vi "Receive Message.vi"(6 "priority":i32, 10 "Async Methods Actor in":refnum<class "Async Methods Actor.lvclass">, 11 "Message in":refnum<class "Message.lvclass">) -> (0 "error out":errorcluster, 2 "Async Actor out":refnum<class "Actor.lvclass">)   [LabVIEW 2023, in "Async Methods Actor.lvlib" / "Async Methods Actor.lvclass"]
doc: "This VI should be overriden ONLY if you are creating a proxy actor for remote transmission. If you are, override this VI to transmit the received message to a new destination, maintaining the given priority."
uses:
  Async Methods Actor.lvclass
  <vilib>/ActorFramework/Message/Message.lvclass
  <vilib>/ActorFramework/Actor/Actor.lvclass
  Async Methods Actor Messages/Async Message/Async Message.lvclass
  <vilib>/ActorFramework/Actor/Actor.lvclass/Actor.ctl
  <vilib>/ActorFramework/Message Enqueuer/Message Enqueuer.lvclass/Message Enqueuer.ctl
  Async Methods Actor.lvclass/Async Methods Actor.ctl
  Async Methods Actor Messages/Async Message/Async Message.lvclass/Async Message.ctl
  <vilib>/ActorFramework/Message Enqueuer/Init from Existing Queue.vi
  Add Async Message to Map.vi
  Async Methods Actor Messages/Async Message/Read Async Call Method.vi
  Async Methods Actor Messages/Async Message/Read VI Refnum Lifetime.vi
  Write Async Message Execution Status Map.vi
  Async Methods Actor Messages/Async Message/Read FQN.vi
  Write Async Message Execution Status Map.vi/3adbf29e-89d7-4ecb-a2bd-8a8b89d527f8.vi
  Get VI FQN.vi
  <vilib>/Utility/LVClass/Get LV Class Path.vi
  <vilib>/ActorFramework/Message Enqueuer/Message Enqueuer.lvclass
  <resource>/AFDebug/AF Debug.lvlib
  C:/Program Files/National Instruments/LabVIEW 2023/vi.lib/ActorFramework/Actor/Actor.lvclass
  C:/Projects/Async Methods Actor/Async Methods Actor/Async Methods Actor/Async Methods Actor.lvclass
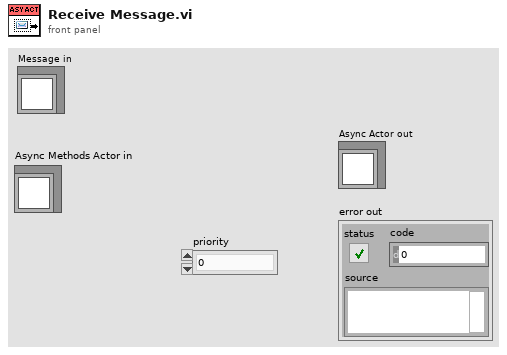
[diagram p1: front panel]
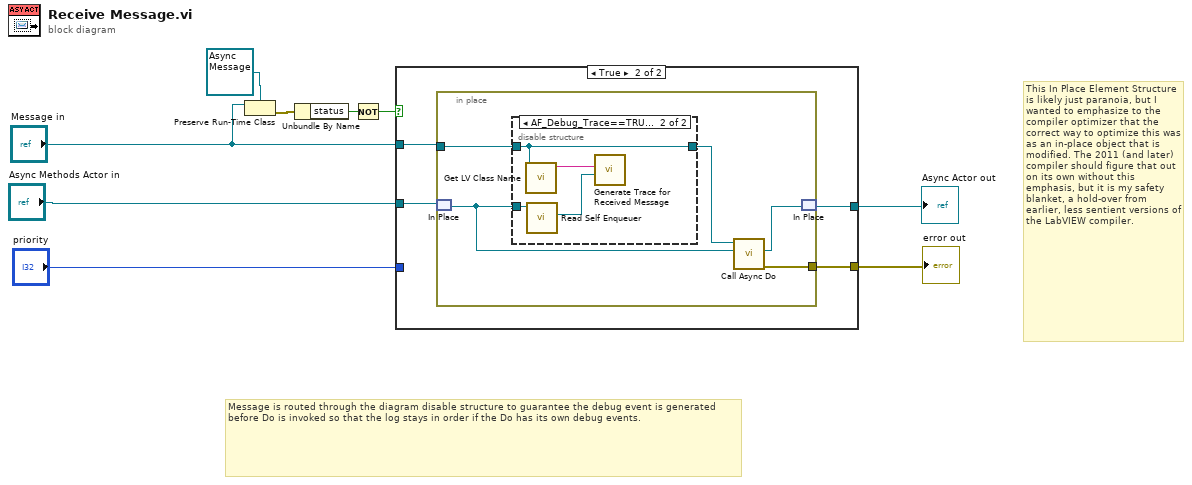
[diagram p0: block diagram]
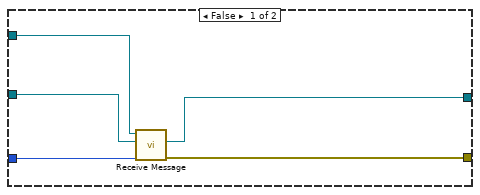
[diagram p2: hidden frame]
diagram:
  # "Message is routed through the diagram disable structure to guarantee the debug event is generated before Do is invoked so that the log stays in order if the Do has its own debug events."
  # "This In Place Element Structure is likely just paranoia, but I wanted to emphasize to the compiler optimizer that the correct way to optimize this was as an in-place object that is modified. The 2011 (and later) compiler should figure that out on its own without this emphasis, but it is my safety blanket, a hold-over from earlier, less sentient versions of the LabVIEW compiler."
  n1 = Preserve Run-Time Class(object in="Message in", 2:refnum<class "Async Message.lvclass"> refnum ("Async Actor.lvlib:Async Message Msg.lvclass")) -> (error out=w2:errorcluster)  [unwired: 1 in, 1 out]
  n2 = Unbundle By Name(w2) -> ("status"=w1:bool)
  n3 = Not(x=w1) -> (.not. x?=w3:bool)
  n4 = case shown="True" w3 {
    tunnel: [w12 w18] -> w9
    tunnel: [w11 w17] -> w8
    tunnel: "Async Methods Actor in" -> [w13 w16]
    tunnel: "Message in" -> [w14 w15]
    tunnel: "priority" -> [w10 _]
    frame False {
      n5 = call-parent "Receive Message.vi"("priority"=w10, "Actor in"=w13, "Message in"=w14) -> ("error out"=w11:errorcluster, "Actor out"=w12:refnum<class "Actor.lvclass">)  [unwired: 7 in]
    }
    frame True {
      n6 = in-place {
        in-place-border: [w23] -> w17
        in-place-border: w15 -> [w21]
        n7 = in-place-match #1(w16) -> (w22:refnum<class "Async Methods Actor.lvclass">)
        n8 = disable-structure shown="AF_Debug_Trace==TRUE" {
          disable-tunnel: w22 -> [_ w28]
          disable-tunnel: w21 -> [w24 w27]
          disable-tunnel: [w24 w27] -> w20
          frame condition #0 {
          }
          frame condition #1 (active) {
            n9 = call <vilib>:"Get LV Class Name.vi"("object"=w27) -> ("class name"=w26:string)  [unwired: 9 in, 1 out]
            n10 = call <vilib>:"Read Self Enqueuer.vi"("Actor"=w28) -> ("Self Enqueuer"=w25:refnum<class "Message Enqueuer.lvclass">)  [unwired: 10 in]
            n11 = call <resource>:"Generate Trace for Received Message.vi"("Actor"=w25, "Message Name"=w26) -> ()  [unwired: 10 in]
          }
        }
        n12 = call "Call Async Do.vi"("Async Methods Actor in"=w22, "Message in"=w20) -> ("error out"=w23:errorcluster, "Async Methods Actor out"=w19:refnum<class "Async Methods Actor.lvclass">)  [unwired: 8 in]
        n13 = in-place-match #1(w19) -> (w18:refnum<class "Async Methods Actor.lvclass">)
      }
    }
  }
  "error out" <- w8
  "Async Actor out" <- w9
